vi "AutoSpeed.vi"(6 "Auto Speed Constants":T3={"Slowing Distance"=0.5, "High Speed"=0.7, "Rampup Time"=250.0, "Low Speed"=0.5, "High Speed (Reverse)"=0.7}, 7 "Encoder Values":T2, 8 "Two Disc Distance":dbl, 9 "Reinitialize":bool, 10 "PID settings":T1, 11 "Target Distance":dbl) -> (0 "Finish":bool, 2 "Backward":bool, 3 "Y axis Speed":dbl, 5 "Two Disc Loading":bool)   [LabVIEW 2013]
uses:
  Auto Speed Constants.ctl
  Encoder Values.ctl
  Robot Global Data.vi
  <vilib>/addons/control/pid/pid.llb/PID (DBL).vi
  <vilib>/addons/control/pid/NI_PID_pid.lvlib
panel:
  out "Current Distance":dbl
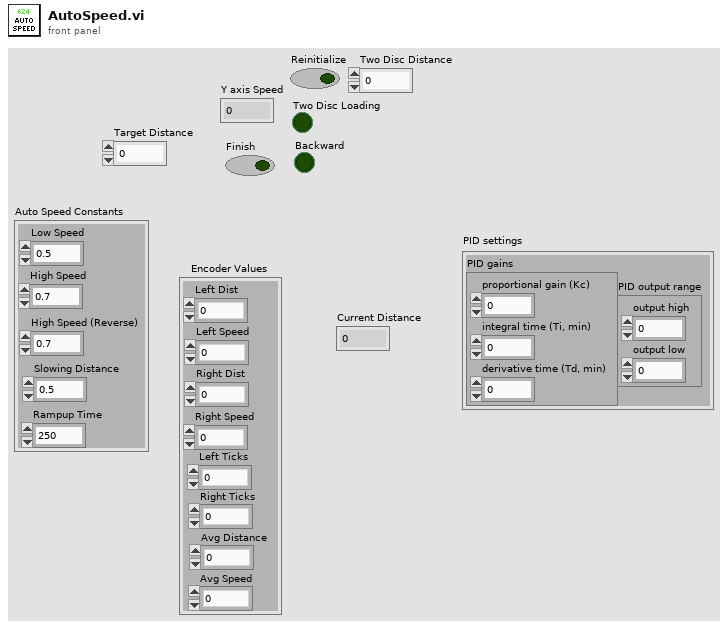
[diagram p1: front panel]
types:
  T1 = cluster{"PID gains":cluster{"proportional gain (Kc)":dbl, "integral time (Ti, min)":dbl, "derivative time (Td, min)":dbl}, "PID output range":cluster{"output high":dbl, "output low":dbl}}
  T2 = typedef "Encoder Values.ctl" = cluster{"Left Dist":dbl, "Left Speed":dbl, "Right Dist":dbl, "Right Speed":dbl, "Left Ticks":dbl, "Right Ticks":dbl, "Avg Distance":dbl, "Avg Speed":dbl}
  T3 = typedef "Auto Speed Constants.ctl" = cluster{"Slowing Distance":dbl, "High Speed":dbl, "Rampup Time":dbl, "Low Speed":dbl, "High Speed (Reverse)":dbl}
  T4 = typedef "UDP Dashboard Packet.ctl" = cluster{"Feed Angle":dbl, "Neutral Angle":dbl, "Autonomous Setpoints":T5, "Auto Shift":T6, "Elevator Angle Offset":dbl, "Potentiometer Angle":cluster{"Pot M":dbl, "Pot B":dbl}, "Shoot Setpoints":cluster{"Vision":T7, "Back Corner":T7, "Front":T7, "Front Corner":T7, "Half Court":T7, "Full Court":T7, "Pyramid":T7}, "Halo Drive":T8, "Auto Speed Constants":T3, "Shooting Delays":cluster{"Unjam On":dbl, "Unjam Off":dbl, "Flipper On":dbl, "Flipper Off":dbl, "Hopper Up":dbl}, "Left Roller Pwr":dbl, "Right Roller Pwr":dbl, "Elevator PID Gains":cluster{"proportional gain (Kc)":dbl, "integral time (Ti, min)":dbl, "derivative time (Td, min)":dbl}, "Elevator PID Output Range":cluster{"output high":dbl, "output low":dbl}, "Elevator Angle Tolerance":dbl, "Toggle Ears Delay":dbl, "Toggle Ears Distance":dbl, "Unjam Servo Angle":dbl, "Auton Steer PID gains":cluster{"proportional gain (Kc)":dbl, "integral time (Ti, min)":dbl, "derivative time (Td, min)":dbl}, "Auton Steer output range":cluster{"output high":dbl, "output low":dbl}, "Auto Reverse Speed":dbl, "Auto Stop Throttle":dbl, "Auto Stop Duration":dbl, "Spin output range":cluster{"output high":dbl, "output low":dbl}, "Spin PID gains":cluster{"proportional gain (Kc)":dbl, "integral time (Ti, min)":dbl, "derivative time (Td, min)":dbl}, "Auto-Center Line":T9, "Auton Distance PID gains Low Gear":cluster{"proportional gain (Kc)":dbl, "integral time (Ti, min)":dbl, "derivative time (Td, min)":dbl}, "Auton Distance output range":cluster{"output high":dbl, "output low":dbl}, "Auton Distance Threshold":dbl, "Auton Velocity Cutoff":dbl, "Auton Distance output range Center Line":cluster{"output high":dbl, "output low":dbl}, "Auton Distance PID gains High Gear":cluster{"proportional gain (Kc)":dbl, "integral time (Ti, min)":dbl, "derivative time (Td, min)":dbl}}
  T5 = typedef "Autonomous Setpoints.ctl" = cluster{"Shoot Angle 1":dbl, "Initial Delay":dbl, "Disc Count 1":dbl, "Shoot Time 1":dbl, "Distance 1":dbl, "Two Disc Distance 1":dbl, "Distance 2":dbl, "Two Disc Distance 2":dbl, "Distance 3":dbl, "Two Disc Distance 3":dbl, "Shoot Angle 3":dbl, "Disc Count 3":dbl, "Shoot Time 3":dbl, "Distance 4":dbl, "Two Disc Distance 4":dbl, "Low Gear":bool, "Shoot 1 Post Delay":dbl}
  T6 = typedef "Auto Shift Settings.ctl" = cluster{"Enabled":bool, "Upshift Speed":dbl, "Downshift Speed":dbl, "Upshift Throttle":dbl, "Turn Power Diff":dbl, "Motor Limit":dbl, "Encoder Limit":dbl}
  T7 = typedef "Shoot Profile.ctl" = cluster{"Pre RPM":dbl, "Main RPM":dbl, "Angle":dbl}
  T8 = typedef "Halo Drive.ctl" = cluster{"Gains":cluster{"Quickturn_Sens_Low":dbl, "Quickturn_Sens_High":dbl, "Speedturn_Sens_Low":dbl, "Speedturn_Sens_High":dbl}, "QuickTurn Const":dbl, "Loading Throttle Limit":dbl}
  T9 = typedef "Autonomous Center Line Setpoints.ctl" = cluster{"Arc Turn x-axis":dbl, "Arc Turn y-axis":dbl, "Arc Turn Distance":dbl, "Distance 1":dbl, "Two Disc Distance 1":dbl, "Distance 2":dbl, "Two Disc Distance 2":dbl, "Spin Angle":dbl, "Spin Angle tolerance":dbl, "Spin y-axis":dbl, "Spin Distance":dbl, "Center Line Enabled":bool, "Distance 3":dbl, "Two Disc Distance 3":dbl, "Spin Angle 2":dbl, "Spin Angle tolerance 2":dbl, "Spin y-axis 2":dbl, "Spin Distance 2":dbl, "Shoot Angle 1":dbl, "Disc Count 1":dbl, "Shoot Time 1":dbl, "Shoot Angle 3":dbl, "Disc Count 3":dbl, "Shoot Time 3":dbl, "Low Gear":bool}
  T10 = cluster{"proportional gain (Kc)":dbl, "integral time (Ti, min)":dbl, "derivative time (Td, min)":dbl}
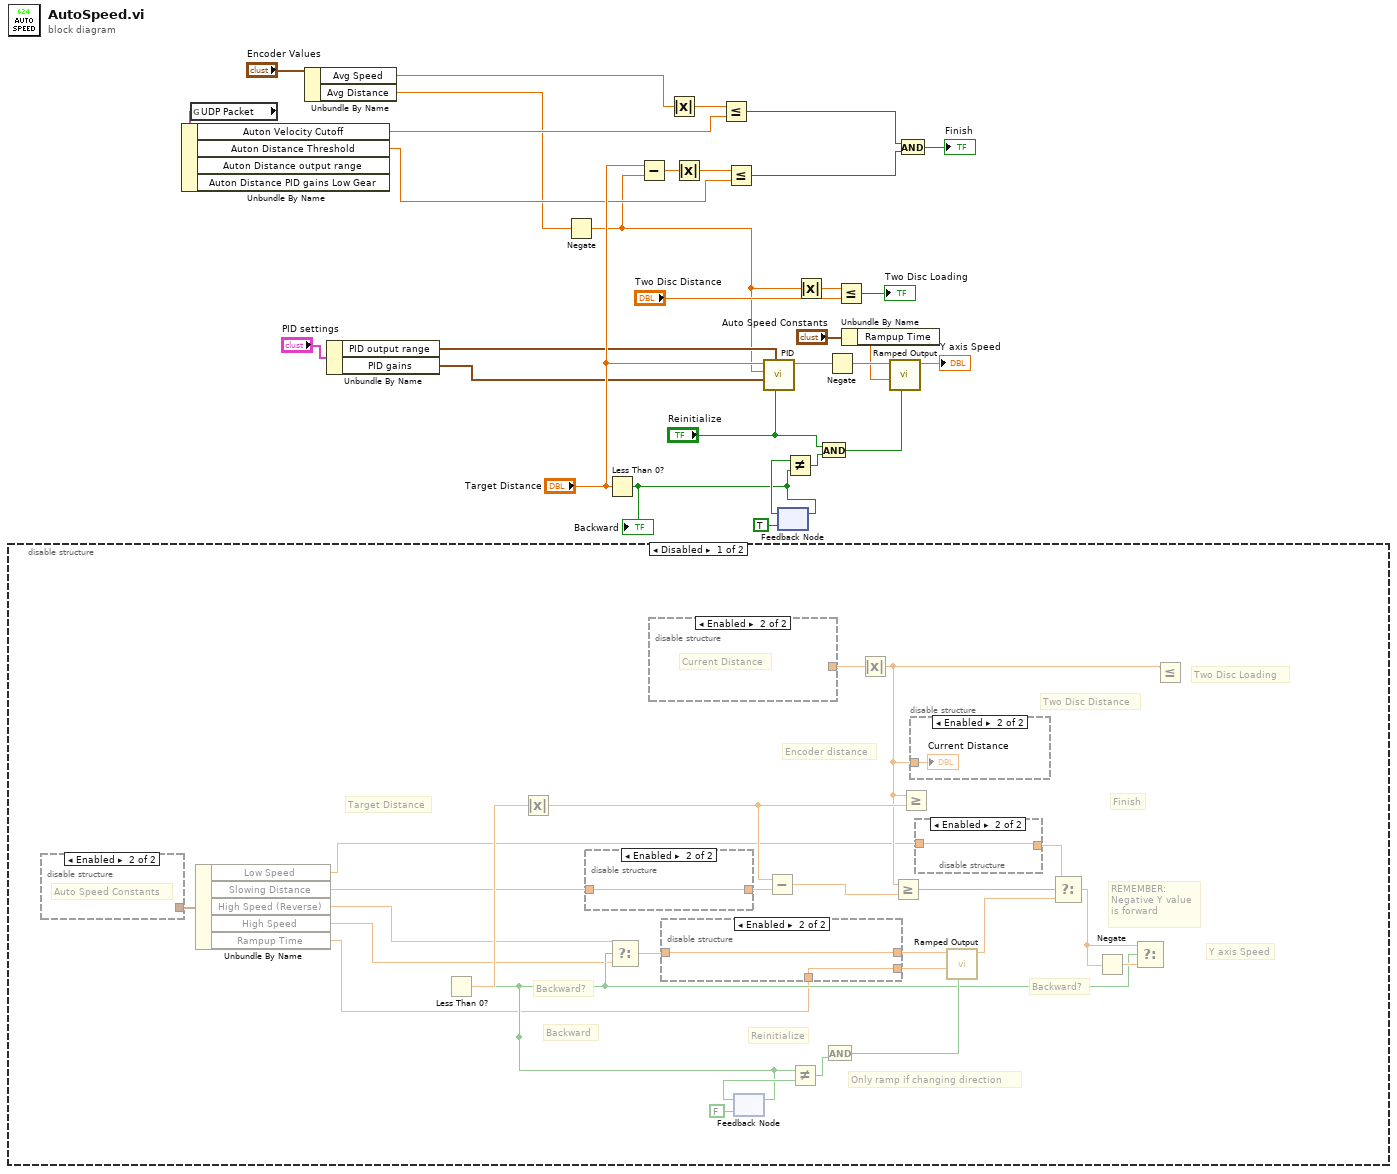
[diagram p0: block diagram]
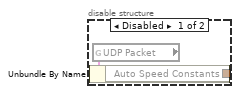
[diagram p2: hidden frame]
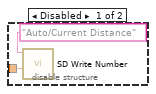
[diagram p3: hidden frame]
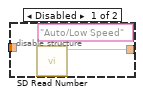
[diagram p4: hidden frame]
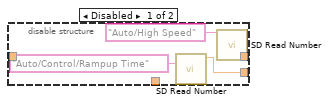
[diagram p5: hidden frame]
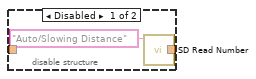
[diagram p6: hidden frame]
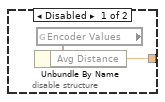
[diagram p7: hidden frame]
diagram:
  n1 = disable-structure shown="Disabled" {
    frame Disabled {
      # "Two Disc Distance"
      # "Reinitialize"
      # "Backward"
      # "Target Distance"
      # "Finish"
      # "Y axis Speed"
      # "Two Disc Loading"
      # "Backward?"
      # "Backward?"
      # "Only ramp if changing direction"
      # "REMEMBER:\nNegative Y value\nis forward"
      # "Encoder distance"
      n2 = disable-structure shown="Enabled" {
        disable-tunnel: [w61 w63] -> w32
        frame Disabled {
          n3 = global read "Robot Global Data.vi" "UDP Packet"() -> (w62:T4)
          n4 = Unbundle By Name(w62) -> ("Auto Speed Constants"=w61:T3)
        }
        frame Enabled {
          # "Auto Speed Constants"
        }
      }
      n5 = Unbundle By Name(w32) -> ("Low Speed"=w37:dbl, "Slowing Distance"=w36:dbl, "High Speed (Reverse)"=w33:dbl, "High Speed"=w34:dbl, "Rampup Time"=w35:dbl)
      n6 = Absolute Value() -> (x=w48:dbl, abs(x)=w55:dbl)
      n7 = Less Than 0?(x=w48) -> (x < 0?=w39:bool)
      n8 = disable-structure shown="Enabled" {
        disable-tunnel: [w77 w78] -> w59
        disable-tunnel: w36 -> [_ w78]
        frame Disabled {
          n9 = call <vilib>:"SD Read Number.vi"("Name"="Auto/Slowing Distance") -> ("Numeric"=w77:dbl)  [unwired: 8 in, 2 out]
        }
        frame Enabled {
        }
      }
      n10 = Select(t=w33, s=w39, f=w34) -> (s? t:f=w38:dbl)
      n11 = disable-structure shown="Enabled" {
        disable-tunnel: [w79 w81] -> w47
        frame Disabled {
          n12 = global read "Robot Global Data.vi" "Encoder Values"() -> (w80:T2)
          n13 = Unbundle By Name(w80) -> ("Avg Distance"=w79:dbl)
        }
        frame Enabled {
          # "Current Distance"
        }
      }
      n14 = disable-structure shown="Enabled" {
        disable-tunnel: [w71 w75] -> w51
        disable-tunnel: [w70 w74] -> w49
        disable-tunnel: w38 -> [_ w75]
        disable-tunnel: w35 -> [_ w74]
        frame Disabled {
          n15 = call <vilib>:"SD Read Number.vi"("Name"="Auto/Control/Rampup Time") -> ("Numeric"=w70:dbl)  [unwired: 8 in, 2 out]
          n16 = call <vilib>:"SD Read Number.vi"("Name"="Auto/High Speed") -> ("Numeric"=w71:dbl)  [unwired: 8 in, 2 out]
        }
        frame Enabled {
        }
      }
      n17 = feedback #1(FALSE) -> (w46:bool)
      n18 = feedback-in #1(w39) -> ()
      n19 = Subtract(x=w55, y=w59) -> (x-y=w60:dbl)
      n20 = Not Equal?(x=w39, y=w46) -> (x != y?=w45:bool)
      n21 = And(y=w45) -> (x .and. y?=w44:bool)  [unwired: 1 in]
      n22 = Absolute Value(x=w47) -> (abs(x)=w42:dbl)
      n23 = Greater Or Equal?(x=w42, y=w60) -> (x >= y?=w57:bool)
      n24 = Greater Or Equal?(x=w42, y=w55) -> (x >= y?=w56:bool)
      n25 = disable-structure shown="Enabled" {
        disable-tunnel: w42 -> [w64 w66]
        frame Disabled {
          n26 = call <vilib>:"SD Write Number.vi"("Numeric"=w64, "Name"="Auto/Current Distance") -> ()  [unwired: 8 in, 2 out]
        }
        frame Enabled {
          "Current Distance" <- w66
        }
      }
      n27 = disable-structure shown="Enabled" {
        disable-tunnel: [w68 w69] -> w58
        disable-tunnel: w37 -> [_ w69]
        frame Disabled {
          n28 = call <vilib>:"SD Read Number.vi"("Name"="Auto/Low Speed") -> ("Numeric"=w68:dbl)  [unwired: 8 in, 2 out]
        }
        frame Enabled {
        }
      }
      n29 = call "Ramped Output.vi"("Reinitialize"=w44, "Rampup Time"=w49, "Base Power"=w51) -> ("Ramped Output"=w50:dbl)  [unwired: 8 in]
      n30 = Select(t=w58, s=w57, f=w50) -> (s? t:f=w52:dbl)
      n31 = Negate(x=w52) -> (-x=w53:dbl)
      n32 = Select(t=w52, s=w39, f=w53) -> (s? t:f=w54:dbl)
      n33 = Less Or Equal?(x=w42) -> (y=w41:dbl, x <= y?=w40:bool)
    }
    frame Enabled {
    }
  }
  n34 = global read "Robot Global Data.vi" "UDP Packet"() -> (w25:T4)
  n35 = Unbundle By Name(w25) -> ("Auton Velocity Cutoff"=w21:dbl, "Auton Distance Threshold"=w24:dbl)  [unwired: 2 out]
  n36 = Unbundle By Name("Encoder Values") -> ("Avg Speed"=w17:dbl, "Avg Distance"=w16:dbl)
  n37 = Unbundle By Name("PID settings") -> ("PID output range"=w4:cluster{"output high":dbl, "output low":dbl}, "PID gains"=w3:T10)
  n38 = Negate(x=w16) -> (-x=w1:dbl)
  n39 = Less Than 0?(x="Target Distance") -> (x < 0?=w8:bool)
  "Backward" <- w8
  n40 = Subtract(x="Target Distance", y=w1) -> (x-y=w28:dbl)
  n41 = Absolute Value(x=w17) -> (abs(x)=w20:dbl)
  n42 = Absolute Value(x=w28) -> (abs(x)=w27:dbl)
  n43 = Less Or Equal?(x=w20, y=w21) -> (x <= y?=w19:bool)
  n44 = Less Or Equal?(x=w27, y=w24) -> (x <= y?=w23:bool)
  n45 = call-poly <vilib>:"PID.vi"("reinitialize? (F)"="Reinitialize", "output range"=w4, "PID gains"=w3, "process variable"=w1, "setpoint"="Target Distance") -> ("output"=w26:dbl)  [unwired: 5 in, 1 out]
  n46 = feedback #2(TRUE) -> (w10:bool)
  n47 = feedback-in #2(w8) -> ()
  n48 = Not Equal?(x=w10, y=w8) -> (x != y?=w9:bool)
  n49 = Absolute Value(x=w1) -> (abs(x)=w2:dbl)
  n50 = And(x="Reinitialize", y=w9) -> (x .and. y?=w6:bool)
  n51 = Negate(x=w26) -> (-x=w15:dbl)
  n52 = Less Or Equal?(x=w2, y="Two Disc Distance") -> (x <= y?=→"Two Disc Loading":bool)
  n53 = Unbundle By Name("Auto Speed Constants") -> ("Rampup Time"=w12:dbl)
  n54 = call "Ramped Output.vi"("Reinitialize"=w6, "Rampup Time"=w12, "Base Power"=w15) -> ("Ramped Output"=→"Y axis Speed":dbl)  [unwired: 8 in]
  n55 = And(x=w19, y=w23) -> (x .and. y?=→"Finish":bool)
